vi "PRL TS Get Real Timestamp.vi"() -> (0 "Time Stamp":timestamp)   [LabVIEW 2012, in "PMU Recorder Light.lvlib"]
uses:
  PMU Recorder Light.lvlib
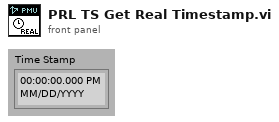
[diagram p1: front panel]
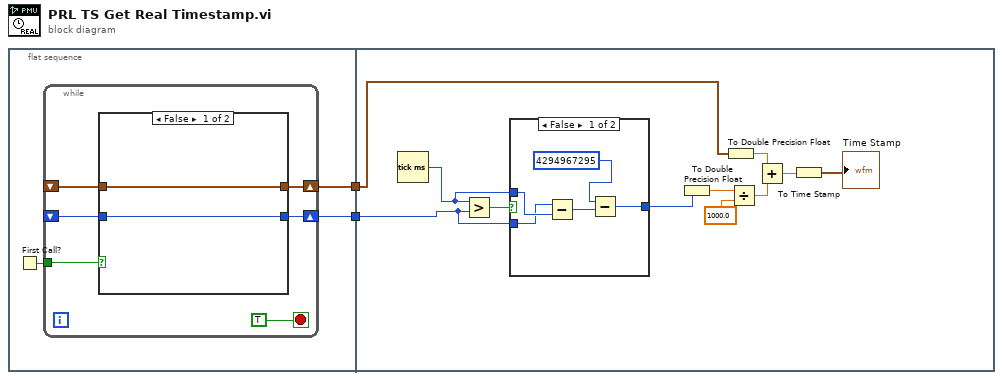
[diagram p0: block diagram]
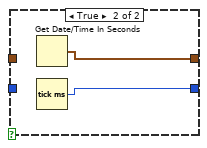
[diagram p2: hidden frame]
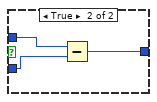
[diagram p3: hidden frame]
diagram:
  n1 = flat-sequence {
    tunnel: [w5] -> w2
    tunnel: [w4] -> w1
    tunnel: w2 -> [w17]
    tunnel: w1 -> [w16]
    frame #0 {
      n2 = First Call?() -> (First Call?: T/F=w3:bool)
      n3 = while {
        shift-right: [w10] -> w5
        shift-left: _ -> [w8]
        shift-right: [w9] -> w4
        shift-left: _ -> [w7]
        tunnel: w3 -> [w6]
        stop <- TRUE stop-if-true
        n4 = case shown="False" w6 {
          tunnel: [w13 w15] -> w10
          tunnel: [w12 w14] -> w9
          tunnel: w8 -> [w13 _]
          tunnel: w7 -> [w12 _]
          frame False {
          }
          frame True {
            n5 = Get Date/Time In Seconds() -> (seconds since 1Jan1904=w15:timestamp)
            n6 = Tick Count (ms)() -> (millisecond timer value=w14:u32)
          }
        }
      }
    }
    frame #1 {
      n7 = Tick Count (ms)() -> (millisecond timer value=w26:u32)
      n8 = Greater?(x=w26, y=w16) -> (0:w24:bool)
      n9 = case shown="False" w24 {
        tunnel: [w27 w32] -> w22
        tunnel: w26 -> [w31 w34]
        tunnel: w16 -> [w30 w33]
        frame False {
          n10 = Subtract(x=w30, y=w31) -> (x-y=w29:u32)
          n11 = Subtract(x=u32 4294967295, y=w29) -> (x-y=w27:u32)
        }
        frame True {
          n12 = Subtract(x=w34, y=w33) -> (x-y=w32:u32)
        }
      }
      n13 = To Double Precision Float(number=w22) -> (double precision float=w25:dbl)
      n14 = To Double Precision Float(number=w17) -> (double precision float=w19:dbl)
      n15 = Divide(x=w25, y=1000.0) -> (x/y=w20:dbl)
      n16 = Add(x=w19, y=w20) -> (x+y=w21:dbl)
      n17 = To Time Stamp(1:w21) -> (0:→"Time Stamp":timestamp)
    }
  }
